vi "HostToFPGA.vi"(8 "Max Count Per Read":i32, 9 "Image in":T1, 10 "Write Timeout (ms)":i32, 11 "Reference in":refnum<k20>) -> (0 "error out":errorcluster, 3 "Image out":T1)   [LabVIEW 2016]
uses:
  <vilib>/vision/Image Controls.llb/IMAQ Image.ctl
  <vilib>/vision/EDVR.llb/IMAQ ImageToEDVR 2D U32.vi
  <vilib>/rvi/errors/niLvFpgaAdjustHostInterfaceError.vi
  <vilib>/rvi/interface/nirviMethod/nirviMethod.xnode
  <vilib>/FPGAPlugInAG/Dynamic/niLvFpga_WriteFifo_Dynamic.vi
  <vilib>/rvi/errors/niLvFpgaMergeErrorWithErrorCode.vi
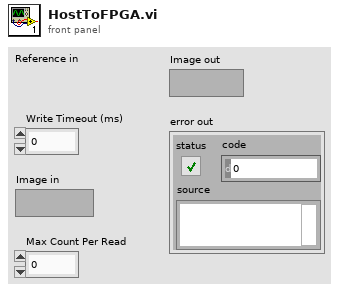
[diagram p1: front panel]
types:
  T1 = typedef "IMAQ Image.ctl" = refnum<image>
  T2 = typedef "Image Type" = u32
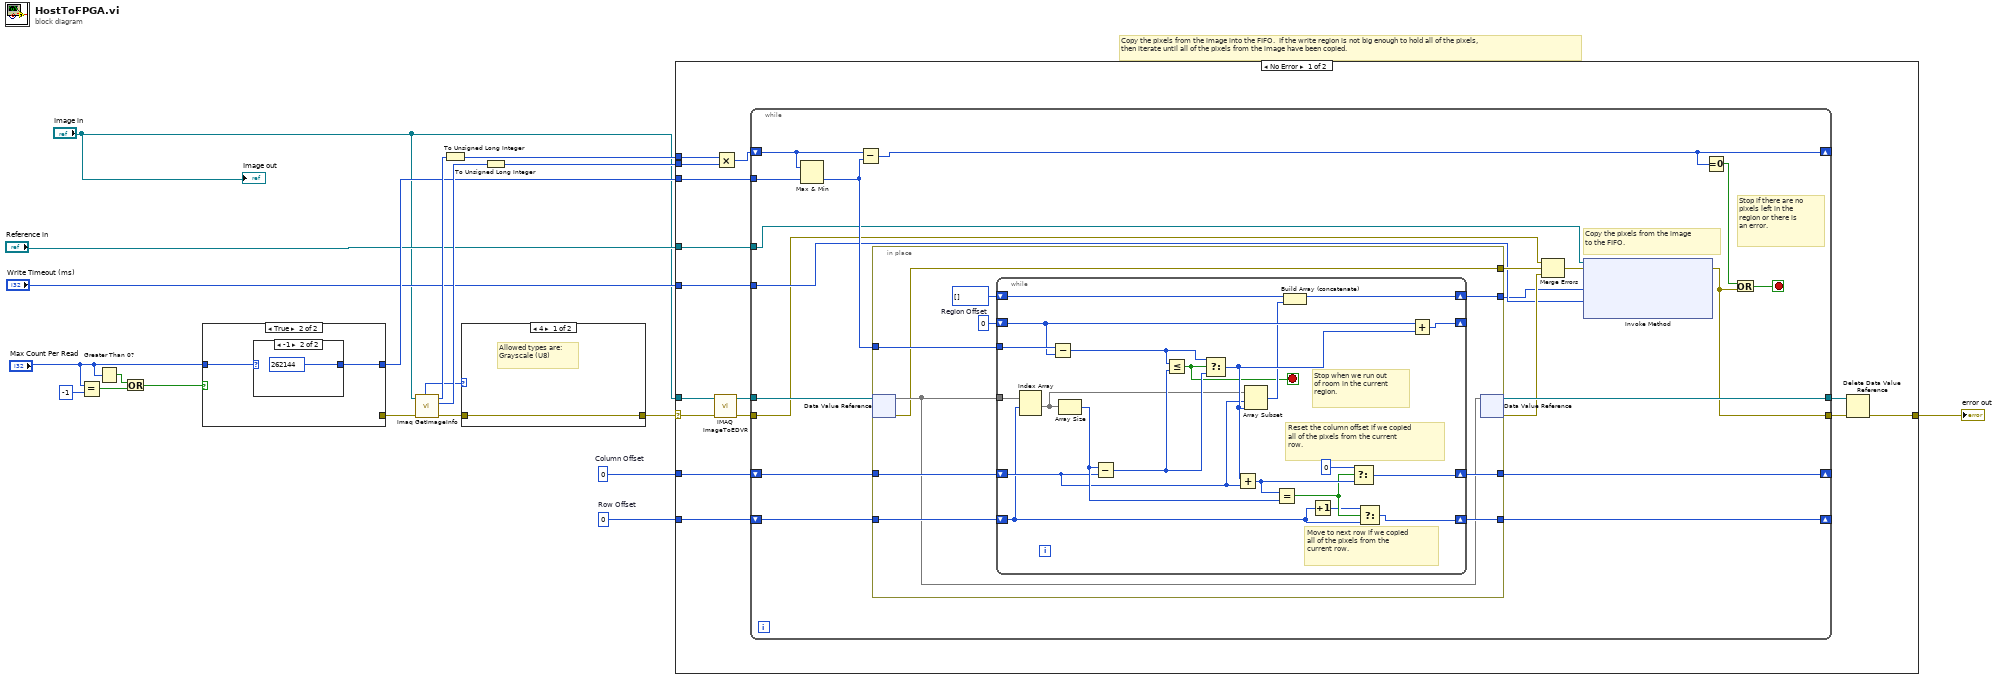
[diagram p0: block diagram]
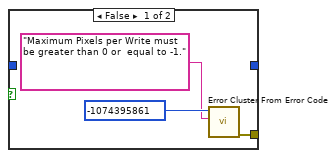
[diagram p2: hidden frame]
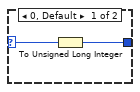
[diagram p3: hidden frame]
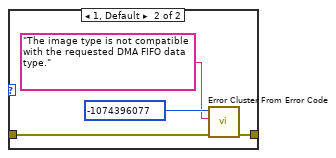
[diagram p5: hidden frame]
diagram:
  w13 = u32 0  # Row Offset
  w12 = u32 0  # Column Offset
  # "Copy the pixels from the image into the FIFO.  If the write region is not big enough to hold all of the pixels,\nthen iterate until all of the pixels from the image have been copied."
  n1 = Equal?(x="Max Count Per Read", y=-1) -> (x = y?=w3:bool)
  n2 = Greater Than 0?(x="Max Count Per Read") -> (x > 0?=w2:bool)
  n3 = Or(x=w2, y=w3) -> (x .or. y?=w4:bool)
  n4 = case shown="True" w4 {
    tunnel: [w21 _] -> w14
    tunnel: "Max Count Per Read" -> [_ w25]
    tunnel: [_ w24] -> w15
    frame False {
      n5 = call <vilib>:"Error Cluster From Error Code.vi"("error message (\"\")"="Maximum Pixels per Write must be greater than 0 or  equal to -1." ("error message (\"\")"), "error code (0)"=-1074395861) -> ("error out"=w21:errorcluster)  [unwired: 7 in]
    }
    frame True {
      n6 = case shown="-1" w25 {
        selector: w25 -> [w27 _]
        tunnel: [w26 u32 262144 ("Maximum Pixels per Write")] -> w24
        frame 0, Default {
          n7 = To Unsigned Long Integer(number=w27) -> (unsigned 32bit integer=w26:u32)
        }
        frame -1 {
        }
      }
    }
  }
  n8 = call "Imaq GetImageInfo"("error in (no error)"=w14, "Image"="Image in") -> ("error out"=w11:errorcluster, "Y Resolution"=w18:i32, "X Resolution"=w17:i32, "Image Type"=w10:T2)  [unwired: 2 in, 4 out]
  n9 = To Unsigned Long Integer(number=w17) -> (unsigned 32bit integer=w19:u32)
  n10 = case shown="4" w10 {
    tunnel: w11 -> [w29 w31]
    tunnel: [w29 w30] -> w16
    frame 4 {
      # "Allowed types are:\nGrayscale (U8)"
    }
    frame 1, Default {
      n11 = call <vilib>:"Error Cluster From Error Code.vi"("error in (no error)"=w31, "error message (\"\")"="The image type is not compatible with the requested DMA FIFO data type." ("error message (\"\")"), "error code (0)"=-1074396077) -> ("error out"=w30:errorcluster)  [unwired: 6 in]
    }
  }
  n12 = To Unsigned Long Integer(number=w18) -> (unsigned 32bit integer=w20:u32)
  n13 = case shown="No Error" w16 {
    selector: w16 -> [w43 w100]
    tunnel: w12 -> [w45 _]
    tunnel: w13 -> [w44 _]
    tunnel: "Reference in" -> [w47 _]
    tunnel: [w41 w100] -> w5
    tunnel: w15 -> [w48 _]
    tunnel: "Write Timeout (ms)" -> [w46 _]
    tunnel: "Image in" -> [w42 _]
    tunnel: w19 -> [w40 _]
    tunnel: w20 -> [w39 _]
    frame No Error {
      n14 = call-poly <vilib>:"IMAQ ImageToEDVR.vi"("error out"=w43, "Image"=w42) -> ("error out"=w37:errorcluster, "EDVR 2D U32"=w38:refnum<data-value>)  [unwired: 7 in, 1 out]
      n15 = Multiply(x=w40, y=w39) -> (x*y=w34:u32)
      n16 = while {
        shift-right: [w62] -> _
        shift-left: w34 -> [w59]
        tunnel: w38 -> [w68]
        shift-right: [w64] -> _
        shift-left: w45 -> [w66]
        shift-right: [w67] -> _
        shift-left: w44 -> [w65]
        tunnel: w47 -> [w49]
        tunnel: [w63] -> w36
        tunnel: [w52] -> w35
        tunnel: w48 -> [w58]
        tunnel: w46 -> [w54]
        tunnel: w37 -> [w50]
        stop <- w61 stop-if-true
        # "Copy the pixels from the image\nto the FIFO."
        # "Stop if there are no\npixels left in the \nregion or there is\nan error."
        n17 = Max & Min(x=w59, y=w58) -> (min(x,y)=w57:u32)  [unwired: 1 out]
        n18 = Subtract(x=w59, y=w57) -> (x-y=w62:u32)
        n19 = in-place {
          in-place-border: w57 -> [w76]
          in-place-border: [w78] -> w67
          in-place-border: w66 -> [w75]
          in-place-border: w65 -> [w73]
          in-place-border: [w74] -> w64
          in-place-border: [w70] -> w56
          in-place-border: [w69] -> w51
          w77 = u32 0  # Region Offset
          n20 = in-place-dvr #1(w68) -> (w72:u32[][], w70:errorcluster)
          n21 = while {
            tunnel: w72 -> [w85]
            shift-right: [w97] -> _
            shift-left: w77 -> [w96]
            tunnel: w76 -> [w99]
            shift-right: [w90] -> w74
            shift-left: w75 -> [w86]
            shift-right: [w80] -> w69
            shift-left: u8[] [] -> [w82]
            shift-right: [w87] -> w78
            shift-left: w73 -> [w83]
            stop <- w79 stop-if-true
            # "Stop when we run out\nof room in the current\nregion."
            # "Reset the column offset if we copied\nall of the pixels from the current\nrow."
            # "Move to next row if we copied\nall of the pixels from the\ncurrent row."
            n22 = Index Array(array=w85, index (row)=w83) -> (element=w84:u32[])  [unwired: 1 in]
            n23 = Subtract(x=w99, y=w96) -> (x-y=w98:u32)
            n24 = Array Size(array=w84) -> (size(s)=w95:i32)
            n25 = Subtract(x=w95, y=w86) -> (x-y=w93:u32)
            n26 = Less Or Equal?(x=w98, y=w93) -> (x <= y?=w79:bool)
            n27 = Select(t=w98, s=w79, f=w93) -> (s? t:f=w94:u32)
            n28 = Add(x=w94, y=w86) -> (x+y=w91:u32)
            n29 = Array Subset(array=w84, index=w86, length=w94) -> (w81:u32[])
            n30 = Equal?(x=w91, y=w95) -> (x = y?=w89:bool)
            n31 = Build Array (concatenate)(w82, w81) -> (w80:u32[])
            n32 = Increment(x=w83) -> (x+1=w88:u32)
            n33 = Select(t=u32 0 ("Elements In Region"), s=w89, f=w91) -> (s? t:f=w90:u32)
            n34 = Select(t=w88, s=w89, f=w83) -> (s? t:f=w87:u32)
            n35 = Add(x=w96, y=w94) -> (x+y=w97:u32)
          }
          n36 = in-place-dvr #1(w72) -> (w63:refnum<data-value>, w55:errorcluster)
        }
        n37 = Merge Errors(w50, w56, w55) -> (w53:errorcluster)
        n38 = xnode "Invoke Method"("FPGA VI Reference In"=w49, "error in"=w53, "Data"=w51, "Timeout (ms)"=w54) -> ("error out"=w52:errorcluster)  [unwired: 2 out]
        n39 = Equal To 0?(x=w62) -> (x = 0?=w60:bool)
        n40 = Or(x=w60, y=w52) -> (x .or. y?=w61:bool)
      }
      n41 = Delete Data Value Reference(data value reference=w36, error in=w35) -> (error out=w41:errorcluster)  [unwired: 1 out]
    }
    frame Error {
    }
  }
  "error out" <- w5
  "Image out" <- "Image in"
